vi "WSVCAP SHL Host TL SPI Write Cycle - Single DUT.vi"(0 "Data Out (Cycle Commands)":string[](array[string]), 5 "Post Command Delay":dbl[](array[numeric]) format="%#.0p s", 11 "error in":errorcluster, 12 "Log (T)":bool=TRUE, 13 "DUT":T1) -> (15 "error out":errorcluster)   [LabVIEW 2012]
uses:
  Type Defs/WSVCAP SHL DUT Number Enum.ctl
  user.lib/Utilities/Type Defs/MISC IO Choice Enum.ctl
panel:
  out "Socket Mask":u16=1 format="%02x"
  out "SPI Data Out":u8[][](array[numeric]) format="%02x"
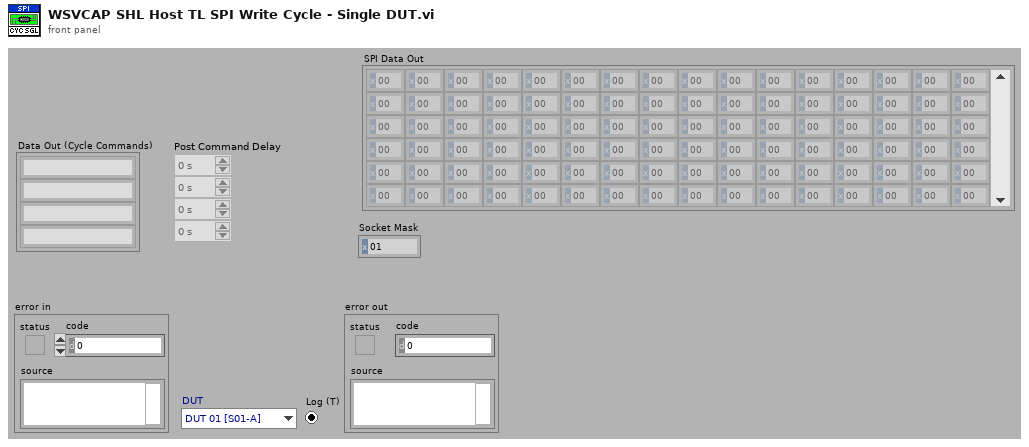
[diagram p1: front panel]
types:
  T1 = typedef "WSVCAP SHL DUT Number Enum.ctl" = enum16{"DUT 01 [S01-A]", "DUT 02 [S02-B]", "DUT 03 [S03-C]", "DUT 04 [S04-D]", "DUT 05 [S05-E]", "DUT 06 [S06-F]", "DUT 07 [S07-G]", "DUT 08 [S08-H]", "DUT 09 [S09-I]", "DUT 10 [S10-J]", "DUT 11 [S11-K]", "DUT 12 [S12-L]", "DUT 13 [S13-M]", "DUT 14 [S14-N]", "DUT 15 [S15-O]", "DUT 16 [S16-P]"}
  T2 = typedef "MISC IO Choice Enum.ctl" = enum16{"Read", "Write"}
  T3 = typedef "WSVCAP SHL Core System Cluster.ctl" = cluster{"Settings":T4, "FPGA Resource":tag, "Online":bool, "I2C Wait Ticks":u32, "SPI Wait Ticks":u32, "RFFE Wait Ticks":u32}
  T4 = typedef "WSVCAP SHL I2C Settings Cluster.ctl" = cluster{"FPGA Resource Name":string, "I2C Slave Address":u8, "I2C Clock Rate (Hz)":dbl, "SPI Clock Rate (Hz)":dbl, "RFFE Slave Address":u8, "RFFE Clock Rate (Hz)":dbl, "Simulate FPGA":bool}
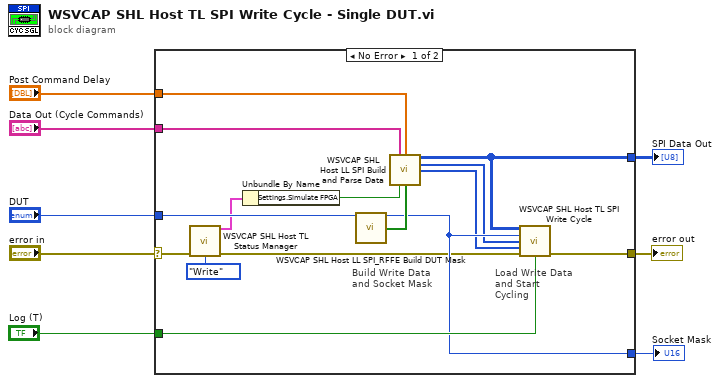
[diagram p0: block diagram]
diagram:
  n1 = case shown="No Error" "error in" {
    selector: "error in" -> [w14 _]
    tunnel: [w16 _] -> w8
    tunnel: [w21 _] -> w6
    tunnel: "DUT" -> [w23 _]
    tunnel: [w19 _] -> w4
    tunnel: "Log (T)" -> [w20 _]
    tunnel: "Post Command Delay" -> [w18 _]
    tunnel: "Data Out (Cycle Commands)" -> [w17 _]
    frame No Error {
      # "Load Write Data and Start Cycling"
      # "Build Write Data and Socket Mask"
      n2 = call "WSVCAP SHL Host TL Status Manager.vi"("error in"=w14, "Operation (Read)"=MISC_IO_Choice_Enum."Write") -> ("System Out"=w12:T3, "error out"=w13:errorcluster)  [unwired: 12 in]
      n3 = Unbundle By Name(w12) -> ("Settings.Simulate FPGA"=w11:bool)
      n4 = call "WSVCAP SHL Host LL SPI_RFFE Build DUT Mask.vi"("DUT"=w23) -> ("Socket Mask [U16]"=w19:u16, "DUT Mask"=w22:bool[])  [unwired: 12 in, 1 out]
      n5 = call "WSVCAP SHL Host LL SPI Build and Parse Data.vi"("Data Out (Cycle Commands)"=w17, "Post Command Delay"=w18, "Simulate FPGA (Cycle Only)"=w11, "DUT Mask (All)"=w22) -> ("SPI Data Out [U8]"=w21:u8[][], "CMD Lengths (Bits)"=w10:u8[], "CMD Delays (Ticks)"=w9:u32[])  [unwired: 8 in, 1 out]
      n6 = call "WSVCAP SHL Host TL SPI Write Cycle.vi"("SPI Data Out"=w21, "Socket Mask"=w19, "Cycle CMD Lengths (bits)"=w10, "Cycle CMD Delay (ticks)"=w9, "error in"=w13, "Log (T)"=w20) -> ("error out"=w16:errorcluster)  [unwired: 9 in]
    }
    frame Error {
    }
  }
  "error out" <- w8
  "SPI Data Out" <- w6
  "Socket Mask" <- w4
